vi "Memory.Pointer.Clear.vi"(8 "error in (no error)":errorcluster, 11 "Pointer in":refnum<class "Memory.Pointer.lvclass">) -> (0 "error out":errorcluster, 3 "Pointer out":refnum<class "Memory.Pointer.lvclass">)   [LabVIEW 2016, in "LabVIEW Memory Manager.lvlib" / "Memory.Pointer.lvclass"]
uses:
  Memory.Pointer.lvclass
  Memory.Pointer.lvclass/Memory.Pointer.ctl
  LabVIEW Memory Manager.lvlib
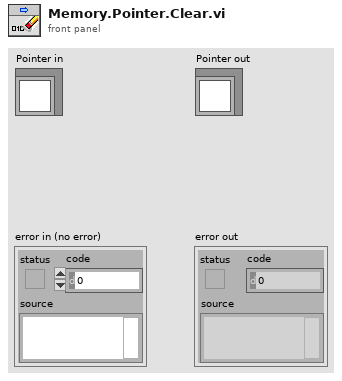
[diagram p1: front panel]
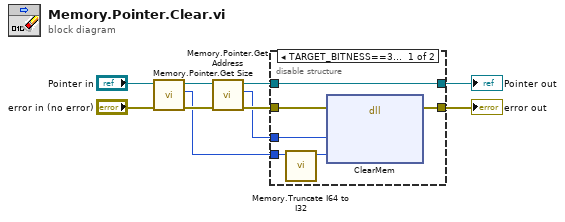
[diagram p0: block diagram]
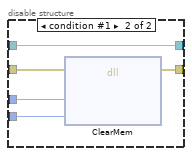
[diagram p2: hidden frame]
diagram:
  n1 = call "Memory.Pointer.Get Size.vi"("error in (no error)"="error in (no error)", "Pointer in"="Pointer in") -> ("error out"=w7:errorcluster, "size"=w6:i64, "Pointer out"=w8:refnum<class "Memory.Pointer.lvclass">)  [unwired: 7 in]
  n2 = call "Memory.Pointer.Get Address.vi"("error in (no error)"=w7, "Pointer in"=w8) -> ("error out"=w5:errorcluster, "address"=w3:u64, "Pointer out"=w2:refnum<class "Memory.Pointer.lvclass">)  [unwired: 7 in]
  n3 = disable-structure shown="TARGET_BITNESS==32, Default" {
    disable-tunnel: w6 -> [w12 w17]
    disable-tunnel: w5 -> [w16 w21]
    disable-tunnel: [w15 w20] -> w4
    disable-tunnel: w3 -> [w14 w19]
    disable-tunnel: w2 -> [w13 w18]
    disable-tunnel: [w13 w18] -> w1
    frame condition #0 (active) {
      n4 = call "Memory.Truncate I64 to I32.vi"("I64"=w12) -> ("truncated I32"=w11:i32)  [unwired: 10 in]
      n5 = dll-call lib="LabVIEW" fn="ClearMem"(error in=w16, "pointer"=w14, "size"=w11) -> (error out=w15:errorcluster)  [unwired: 5 in, 1 out]
    }
    frame condition #1 {
      n6 = dll-call lib="LabVIEW" fn="ClearMem"(error in=w21, "pointer"=w19, "size"=w17) -> (error out=w20:errorcluster)  [unwired: 5 in, 1 out]
    }
  }
  "error out" <- w4
  "Pointer out" <- w1
